vi "SSC DCPower Get Power Line Frequencies.vi"(0 "DCPower SSC in":T1[](array[typedef]), 11 "error in":errorcluster) -> (4 "DCPower SSC out":T1[](array[typedef]), 6 "Configured Power Line Frequencies (Hz)":dbl[](array[numeric]) format="%#_6p", 15 "error out":errorcluster)   [LabVIEW 2019]
doc: "This VI gets the configured power line frequency for the sessions."
uses:
  SSC DCPower.ctl
  SSC DCPower Debug Global.vi
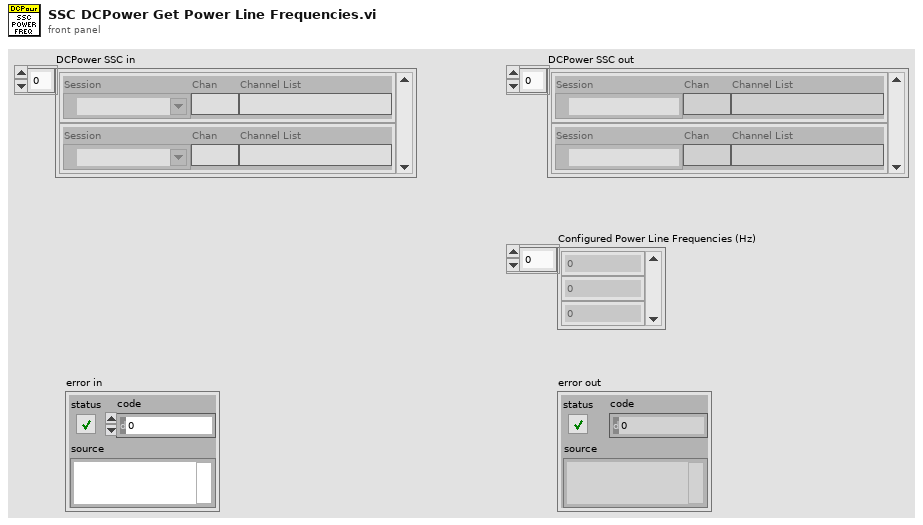
[diagram p1: front panel]
types:
  T1 = typedef "SSC DCPower.ctl" = cluster{"Session":refnum<k15>, "Chan":string, "Channel List":string}
  T2 = typedef "niDCPower Power Line Frequency.ctl" = dbl
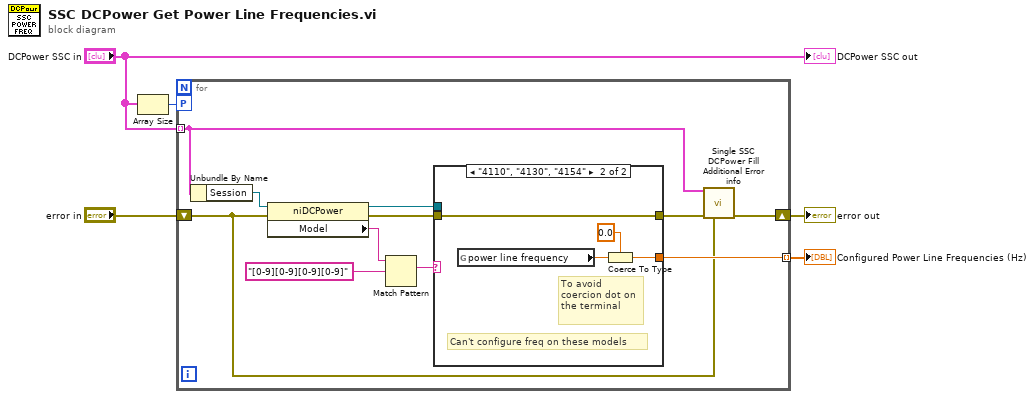
[diagram p0: block diagram]
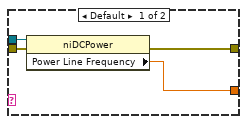
[diagram p2: hidden frame]
diagram:
  n1 = Array Size(array="DCPower SSC in") -> (size(s)=w3:i32)
  n2 = for {
    tunnel: "DCPower SSC in" -> [w7] mode=indexing
    workers-P: w3 -> [_]
    shift-right: [w8] -> w5
    shift-left: "error in" -> [w6]
    tunnel: [w9] -> w1 mode=indexing
    n3 = Unbundle By Name(w7) -> ("Session"=w14:refnum<k15>)
    n4 = property class="niDCPower"(reference=w14, error in=w6) -> (reference out=w13:refnum<k15>, error out=w15:errorcluster, "Model"=w11:string)
    n5 = Match Pattern(string=w11, regular expression="[0-9][0-9][0-9][0-9]") -> (match substring=w10:string)  [unwired: 1 in, 3 out]
    n6 = case shown="\"4110\", \"4130\", \"4154\"" w10 {
      tunnel: [w20 w24] -> w16
      tunnel: w15 -> [w19 w24]
      tunnel: w13 -> [w18 _]
      tunnel: [w17 w21] -> w9
      frame Default {
        n7 = property class="niDCPower"(reference=w18, error in=w19) -> (error out=w20:errorcluster, "Power Line Frequency"=w17:dbl)  [unwired: 1 out]
      }
      frame "4110", "4130", "4154" {
        # "To avoid coercion dot on the terminal"
        # "Can't configure freq on these models"
        n8 = global read "SSC DCPower Debug Global.vi" "power line frequency"() -> (w22:T2)
        n9 = Coerce To Type(0:w22, 1:0.0) -> (2:w21:dbl)
      }
    }
    n10 = call "Single SSC DCPower Fill Additional Error info.vi"("DCPower SSC in"=w7, "error in"=w16, "previous error in"=w6) -> ("error out"=w8:errorcluster)  [unwired: 12 in]
  }
  "Configured Power Line Frequencies (Hz)" <- w1
  "error out" <- w5
  "DCPower SSC out" <- "DCPower SSC in"
